vi "Save Recipe as XML.vi"(8 "error in (no error)":errorcluster, 10 "Path":path, 11 "Process Settings.lvclass":refnum<class "Process Settings.lvclass">) -> (0 "error out":errorcluster)   [LabVIEW 2017, in "Process Settings.lvclass"]
uses:
  Process Settings.lvclass
  <vilib>/Utility/xml.llb/Write to XML File(string).vi
panel:
  out "Process Settings.lvclass":refnum<class "Process Settings.lvclass">
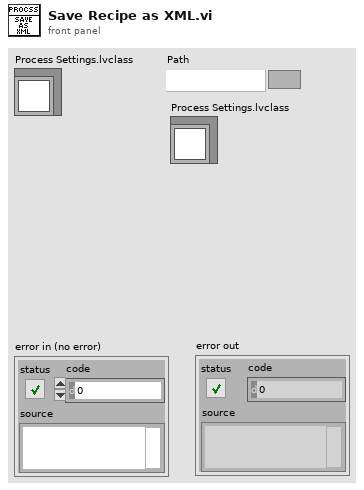
[diagram p1: front panel]
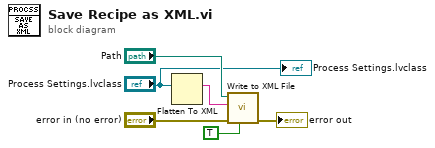
[diagram p0: block diagram]
diagram:
  n1 = Flatten To XML(anything="Process Settings.lvclass") -> (xml string=w5:string)
  n2 = call-poly <vilib>:"Write to XML File.vi"("Standalone? (T)"=TRUE, "error in (no error)"="error in (no error)", "XML Input"=w5, "XML File Path"="Path") -> ("error out"=→"error out":errorcluster)  [unwired: 5 in, 2 out]
  "Process Settings.lvclass" <- "Process Settings.lvclass"
